vi "Write Search.vi"(10 "Search":refnum<class "Search.lvclass">, 11 "ProjectItem in":refnum<class "ProjectItem.lvclass">) -> (3 "ProjectItem out":refnum<class "ProjectItem.lvclass">)   [LabVIEW 2016, in "ProjectItem.lvclass"]
uses:
  ProjectItem.lvclass
  Search/Search.lvclass
  ProjectItem.lvclass/ProjectItem.ctl
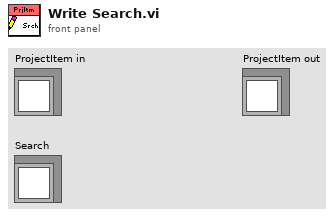
[diagram p1: front panel]
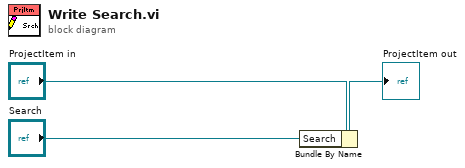
[diagram p0: block diagram]
diagram:
  n1 = Bundle By Name(cluster="ProjectItem in", "Search"="Search") -> (→"ProjectItem out":refnum<class "ProjectItem.lvclass">)
